vi "Trapezoid Quadrature.vi"(10 "Array":dbl[](array[numeric]), 11 "Time":dbl[](array[numeric])) -> (3 "Result":dbl[](array[numeric]))   [LabVIEW 2020]
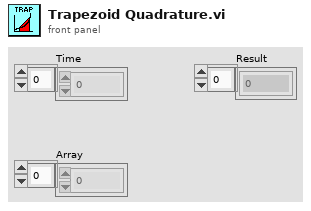
[diagram p1: front panel]
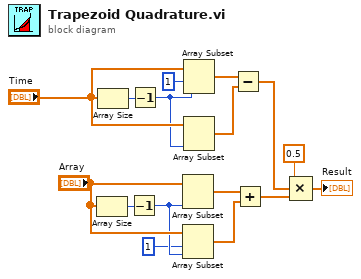
[diagram p0: block diagram]
diagram:
  n1 = Array Size(array="Array") -> (size(s)=w2:i32)
  n2 = Array Size(array="Time") -> (size(s)=w9:i32)
  n3 = Decrement(x=w2) -> (x-1=w4:i32)
  n4 = Decrement(x=w9) -> (x-1=w10:i32)
  n5 = Array Subset(array="Array", length=w4) -> (w6:dbl[])  [unwired: 1 in]
  n6 = Array Subset(array="Array", index=1, length=w4) -> (w7:dbl[])
  n7 = Array Subset(array="Time", index=1, length=w10) -> (w13:dbl[])
  n8 = Array Subset(array="Time", length=w10) -> (w14:dbl[])  [unwired: 1 in]
  n9 = Subtract(x=w13, y=w14) -> (x-y=w15:dbl[])
  n10 = Add(x=w6, y=w7) -> (x+y=w8:dbl[])
  n11 = Compound Arithmetic op=MULTIPLY(0.5 ("Numeric"), w15, w8) -> (→"Result":dbl[])
